vi "BATTERY MAX ENERGY VI.vi"(0 "unsigned byte array[7]":u8, 1 "unsigned byte array[6]":u8, 2 "unsigned byte array[5]":u8, 3 "unsigned byte array[1]":u8, 5 "unsigned byte array[8]":u8, 7 "Numeric 9":dbl, 9 "Numeric 8":dbl, 11 "Numeric 10":dbl, 12 "Boolean":bool, 13 "Numeric 7":dbl, 14 "Numeric 6":dbl) -> (4 "Numeric 4":dbl, 6 "Numeric 3":dbl, 8 "Numeric 2":dbl, 10 "Numeric":dbl, 15 "Numeric 5":dbl)   [LabVIEW 2016]
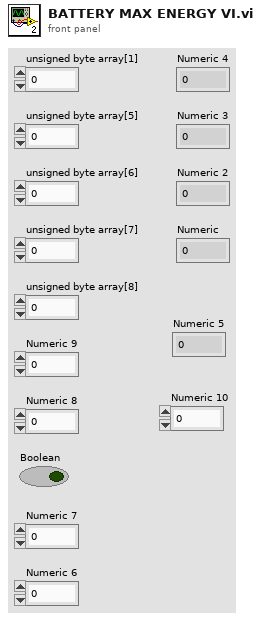
[diagram p1: front panel]
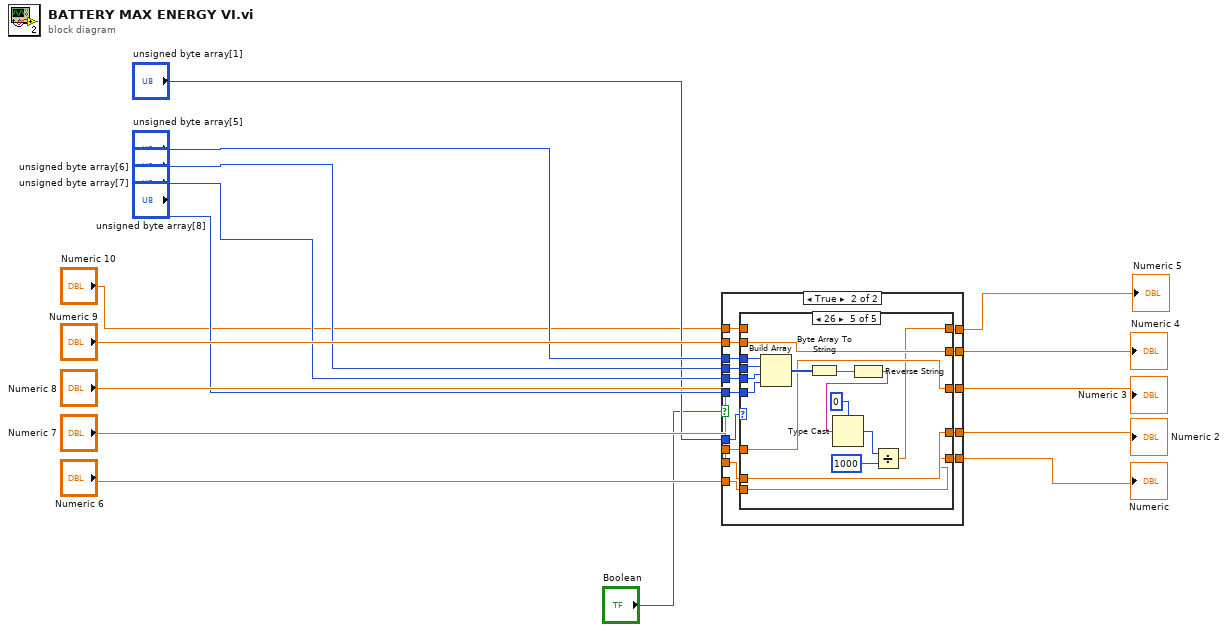
[diagram p0: block diagram]
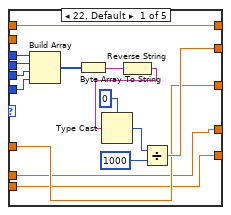
[diagram p3: hidden frame]
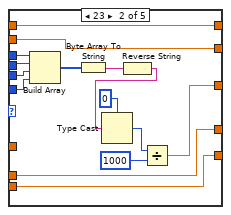
[diagram p4: hidden frame]
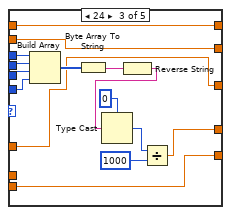
[diagram p5: hidden frame]
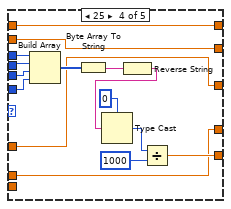
[diagram p6: hidden frame]
diagram:
  n1 = case shown="True" "Boolean" {
    tunnel: "unsigned byte array[5]" -> [_ w36]
    tunnel: "unsigned byte array[6]" -> [_ w35]
    tunnel: "unsigned byte array[7]" -> [_ w34]
    tunnel: "unsigned byte array[8]" -> [_ w33]
    tunnel: "unsigned byte array[1]" -> [_ w32]
    tunnel: [w21 w31] -> w13
    tunnel: [w20 w30] -> w14
    tunnel: [w19 w29] -> w15
    tunnel: [w18 w28] -> w16
    tunnel: "Numeric 9" -> [w21 w24]
    tunnel: "Numeric 8" -> [w20 w27]
    tunnel: "Numeric 7" -> [w19 w26]
    tunnel: "Numeric 6" -> [w18 w25]
    tunnel: [w17 w22] -> w1
    tunnel: "Numeric 10" -> [w17 w23]
    frame False {
    }
    frame True {
      n2 = case shown="26" w32 {
        tunnel: w36 -> [w46 w60 w76 w91 w106]
        tunnel: w35 -> [w45 w59 w75 w90 w105]
        tunnel: w34 -> [w44 w58 w74 w89 w104]
        tunnel: w33 -> [w43 w57 w73 w88 w103]
        tunnel: [w41 w55 w70 w85 w101] -> w31
        tunnel: [w40 w56 w69 w84 w100] -> w30
        tunnel: [w39 w54 w71 w83 w99] -> w29
        tunnel: [w38 w53 w68 w86 w98] -> w28
        tunnel: w27 -> [w40 _ w69 w84 w100]
        tunnel: w26 -> [w39 w54 _ w83 w99]
        tunnel: w25 -> [w38 w53 w68 _ w98]
        tunnel: w24 -> [_ w55 w70 w85 w101]
        tunnel: w23 -> [w37 w52 w67 w82 _]
        tunnel: [w37 w52 w67 w82 w97] -> w22
        frame 22, Default {
          n3 = Build Array(w46, w45, w44, w43) -> (w42:u8[])
          n4 = Byte Array To String(unsigned byte array=w42) -> (string=w47:string)
          n5 = Reverse String(1:w47) -> (0:w51:string)
          n6 = Type Cast(type=0, x=w51) -> (*(type *) &x=w49:i32)
          n7 = Divide(x=w49, y=1000) -> (x/y=w41:dbl)
        }
        frame 23 {
          n8 = Build Array(w60, w59, w58, w57) -> (w61:u8[])
          n9 = Byte Array To String(unsigned byte array=w61) -> (string=w62:string)
          n10 = Reverse String(1:w62) -> (0:w66:string)
          n11 = Type Cast(type=0, x=w66) -> (*(type *) &x=w64:i32)
          n12 = Divide(x=w64, y=1000) -> (x/y=w56:dbl)
        }
        frame 24 {
          n13 = Build Array(w76, w75, w74, w73) -> (w72:u8[])
          n14 = Byte Array To String(unsigned byte array=w72) -> (string=w77:string)
          n15 = Reverse String(1:w77) -> (0:w81:string)
          n16 = Type Cast(type=0, x=w81) -> (*(type *) &x=w79:i32)
          n17 = Divide(x=w79, y=1000) -> (x/y=w71:dbl)
        }
        frame 25 {
          n18 = Build Array(w91, w90, w89, w88) -> (w87:u8[])
          n19 = Byte Array To String(unsigned byte array=w87) -> (string=w92:string)
          n20 = Reverse String(1:w92) -> (0:w96:string)
          n21 = Type Cast(type=0, x=w96) -> (*(type *) &x=w94:i32)
          n22 = Divide(x=w94, y=1000) -> (x/y=w86:dbl)
        }
        frame 26 {
          n23 = Build Array(w106, w105, w104, w103) -> (w102:u8[])
          n24 = Byte Array To String(unsigned byte array=w102) -> (string=w107:string)
          n25 = Reverse String(1:w107) -> (0:w111:string)
          n26 = Type Cast(type=0, x=w111) -> (*(type *) &x=w109:i32)
          n27 = Divide(x=w109, y=1000) -> (x/y=w97:dbl)
        }
      }
    }
  }
  "Numeric" <- w16
  "Numeric 2" <- w15
  "Numeric 3" <- w14
  "Numeric 4" <- w13
  "Numeric 5" <- w1
